vi "Build command substring_C-887.vi"(0 "System no.":i32=1 min=1 max=4 step=1, 2 "Affected axes":string[](array[string]), 3 "Parameters":dbl[](array[numeric]) format="%.8f", 4 "No. of digits":i16=4, 6 "Parameters (hex)":u32[](array[numeric]) format="%.0x", 7 "Parameter no. format \n(Decimal: FALSE)":bool, 9 "With space?":bool) -> (14 "Command substring":string)   [LabVIEW 2020]
doc: "This VI builds a command substring by combining axis identifier and parameter. If parameter no. is in decimal format, use Parameters input, for hexadecimal parameter numbers use Parameters (hex) input and switch Parameter no. format to TRUE. Do not mix decimal and hex. parameter numbers in one call. No. of digits is the number of digits after the decimal point in the parameter value(s) that will be sent.\nExample: For Affected axes = A; B, Parameters = 1.2342; 2.3 and No. of digits = 3 the resulting string is \"SpaceA1.234SpaceB2.300\"."
panel:
  # "This vi builds a command substring by combining axis identifier and parameter. If parameter no. is in \ndecimal format, use \"Parameters\" input, for hexadecimal parameter numbers use \"Parameters (hex)\" \ninput and switch \"Parameter no. format\"  to TRUE. Do not mix decimal and hex. parameter numbers in one call."
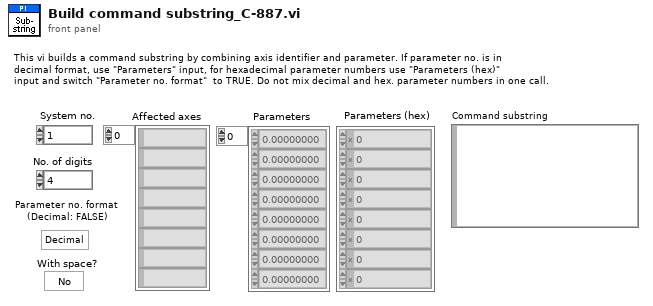
[diagram p1: front panel]
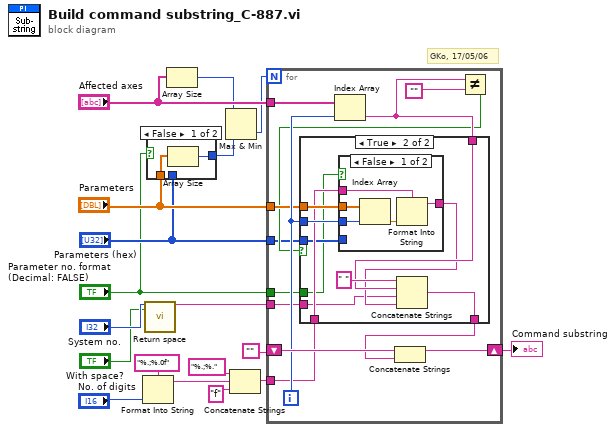
[diagram p0: block diagram]
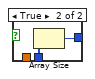
[diagram p2: hidden frame]
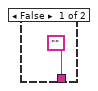
[diagram p3: hidden frame]
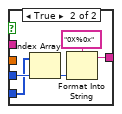
[diagram p4: hidden frame]
diagram:
  # "GKo, 17/05/06"
  n1 = Format Into String(format string="%.;%.0f" ("Format String"), "No. of digits") -> (resulting string=w2:string)  [unwired: 2 in, 1 out]
  n2 = call "Return space.vi"("System no."="System no.", "With space?"="With space?") -> ("String out"=w8:string)  [unwired: 17 out]
  n3 = case shown="False" "Parameter no. format \n(Decimal: FALSE)" {
    tunnel: "Parameters" -> [w20 _]
    tunnel: [w19 w22] -> w14
    tunnel: "Parameters (hex)" -> [_ w21]
    frame False {
      n4 = Array Size(array=w20) -> (size(s)=w19:i32)
    }
    frame True {
      n5 = Array Size(array=w21) -> (size(s)=w22:i32)
    }
  }
  n6 = Array Size(array="Affected axes") -> (size(s)=w13:i32)
  n7 = Max & Min(x=w13, y=w14) -> (min(x,y)=w12:i32)  [unwired: 1 out]
  n8 = Concatenate Strings("%.;%." ("Format String"), w2, "f" ("Format String")) -> (w5:string)
  n9 = for {
    N: w12 -> [_]
    shift-right: [w34] -> w17
    shift-left: "" -> [w35]
    tunnel: "Parameters" -> [w31]
    tunnel: w5 -> [w30]
    tunnel: "Affected axes" -> [w29]
    tunnel: "Parameters (hex)" -> [w25]
    tunnel: "Parameter no. format \n(Decimal: FALSE)" -> [w24]
    tunnel: w8 -> [w23]
    i -> [w32]
    n10 = Index Array(array=w29, index=w32) -> (element=w28:string)
    n11 = Not Equal?(x=w28, y="") -> (x != y?=w26:bool)
    n12 = case shown="True" w26 {
      tunnel: ["" w46] -> w33
      tunnel: w32 -> [_ w45]
      tunnel: w31 -> [_ w44]
      tunnel: w30 -> [_ w43]
      tunnel: w28 -> [_ w41]
      tunnel: w25 -> [_ w40]
      tunnel: w24 -> [_ w39]
      tunnel: w23 -> [_ w37]
      frame False {
      }
      frame True {
        n13 = case shown="False" w39 {
          tunnel: w45 -> [w51 w56]
          tunnel: w44 -> [w50 _]
          tunnel: w43 -> [w49 _]
          tunnel: [w47 w54] -> w38
          tunnel: w40 -> [_ w53]
          frame False {
            n14 = Index Array(array=w50, index=w51) -> (element=w48:dbl)
            n15 = Format Into String(format string=w49, w48) -> (resulting string=w47:string)  [unwired: 2 in, 1 out]
          }
          frame True {
            n16 = Index Array(array=w53, index=w56) -> (element=w55:u32)
            n17 = Format Into String(format string="0X%0x" ("Format String"), w55) -> (resulting string=w54:string)  [unwired: 2 in, 1 out]
          }
        }
        n18 = Concatenate Strings(" " ("Substring"), w41, w37, w38) -> (w46:string)
      }
    }
    n19 = Concatenate Strings(w35, w33) -> (w34:string)
  }
  "Command substring" <- w17
